vi "SystemCheckState.vi"(7 "error in (no error)":errorcluster, 9 "State in":T1, 10 "Actual Start [i]":i64) -> (0 "error out":errorcluster, 2 "Cluster":T2, 3 "State Out":T1)   [LabVIEW 2018]
uses:
  Type_Def/Type_Def Actuator Controls.ctl
  Type_Def/Type_Def ControlState.ctl
panel:
  out "Numeric":i64
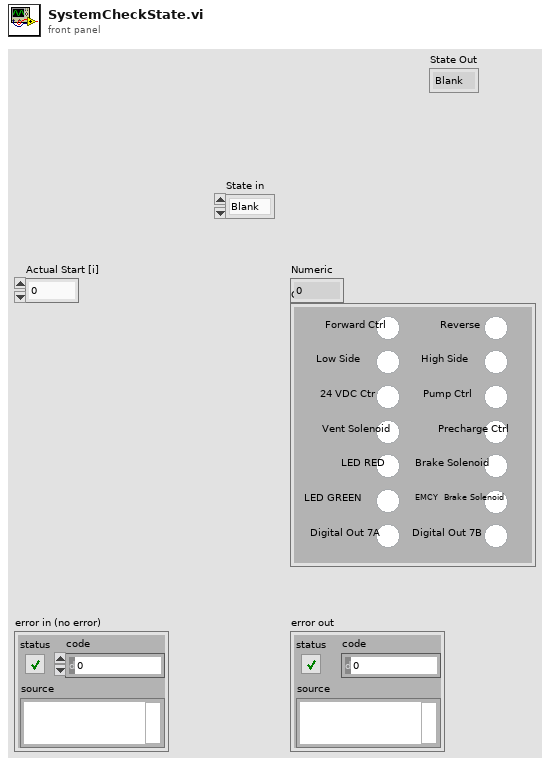
[diagram p1: front panel]
types:
  T1 = typedef "Type_Def ControlState.ctl" = enum16{"Blank", "Systems Check", "Idle", "Ready", "Pushing", "CrawlingPrecharge", "Braking", "Fault", "Boot Up", "Crawling", "Shutdown", "Service Push", "Service Wait", "Vent", "Precharge"}
  T2 = typedef "Type_Def Actuator Controls.ctl" = cluster{"Reverse ":bool, "Precharge Ctrl":bool, "Pump Ctrl":bool, "24 VDC Ctr":bool, "Vent Solenoid":bool, "Brake Solenoid":bool, "EMCY  Brake Solenoid":bool, "Digital Out 7B ":bool, "Forward Ctrl":bool, " Low Side":bool, "High Side":bool, "LED RED":bool, "LED GREEN":bool, " Digital Out 7A":bool}
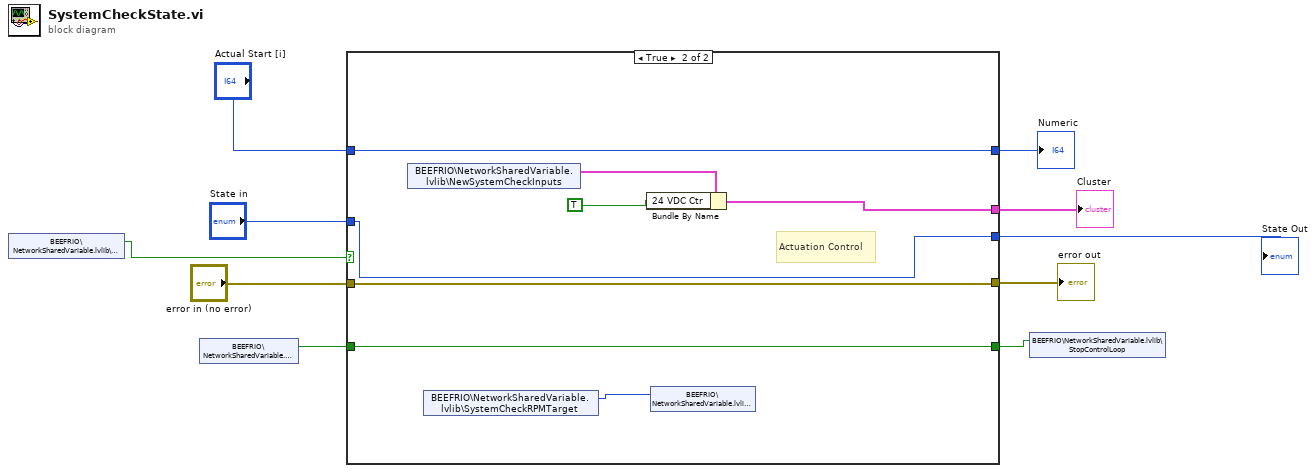
[diagram p0: block diagram]
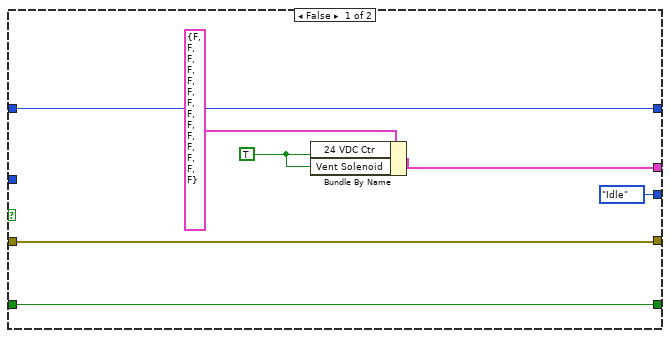
[diagram p2: hidden frame]
diagram:
  n1 = shared-variable "BEEFRIO\\NetworkSharedVariable.lvlib\\SystemCheck"() -> (w2:bool)  [unwired: 1 in, 1 out]
  n2 = shared-variable "BEEFRIO\\NetworkSharedVariable.lvlib\\Shutdown"() -> (w5:bool)  [unwired: 1 in, 1 out]
  n3 = case shown="True" w2 {
    tunnel: [w17 w23] -> w10
    tunnel: "Actual Start [i]" -> [w17 w23]
    tunnel: [w16 w20] -> w8
    tunnel: "error in (no error)" -> [w16 w20]
    tunnel: [w15 w21] -> w6
    tunnel: w5 -> [w15 w21]
    tunnel: [Type_Def_ControlState."Idle" ("Enum in") w22] -> w4
    tunnel: "State in" -> [_ w22]
    tunnel: [w12 w19] -> w1
    frame False {
      w13 = TRUE
      n4 = Bundle By Name(cluster=T2 {"Reverse "=FALSE, "Precharge Ctrl"=FALSE, "Pump Ctrl"=FALSE, "24 VDC Ctr"=FALSE, "Vent Solenoid"=FALSE, "Brake Solenoid"=FALSE, "EMCY  Brake Solenoid"=FALSE, "Digital Out 7B "=FALSE, "Forward Ctrl"=FALSE, " Low Side"=FALSE, "High Side"=FALSE, "LED RED"=FALSE, "LED GREEN"=FALSE, " Digital Out 7A"=FALSE} ("Cluster 2"), "24 VDC Ctr"=w13, "Vent Solenoid"=w13) -> (w12:T2)
    }
    frame True {
      # "Actuation Control"
      n5 = shared-variable "BEEFRIO\\NetworkSharedVariable.lvlib\\NewSystemCheckInputs"() -> (w25:T2)  [unwired: 1 in, 1 out]
      n6 = shared-variable "BEEFRIO\\NetworkSharedVariable.lvlib\\SystemCheckRPMTarget"() -> (w18:i16)  [unwired: 1 in, 1 out]
      n7 = Bundle By Name(cluster=w25, "24 VDC Ctr"=TRUE) -> (w19:T2)
      n8 = shared-variable "BEEFRIO\\NetworkSharedVariable.lvlib\\driveTarget"(w18) -> ()  [unwired: 1 in, 1 out]
    }
  }
  "error out" <- w8
  "Numeric" <- w10
  "State Out" <- w4
  "Cluster" <- w1
  n9 = shared-variable "BEEFRIO\\NetworkSharedVariable.lvlib\\StopControlLoop"(w6) -> ()  [unwired: 1 in, 1 out]
